vi "FTW-Container-Value-EXT.vi"(0 "JSON":refnum<class "FTW-Container.lvclass">, 11 "error in":errorcluster) -> (4 "JSON out":refnum<class "FTW-Container.lvclass">, 8 "Value":ext, 15 "error out":errorcluster)   [LabVIEW 2015, in "FTW-Container.lvclass"]
uses:
  FTW-Container.lvclass
  FTW-Container.lvclass/FTW-Container.ctl
  <vilib>/Utility/Data Type/NI_Data Type.lvlib
panel:
  # "Inputs"
  # "Outputs"
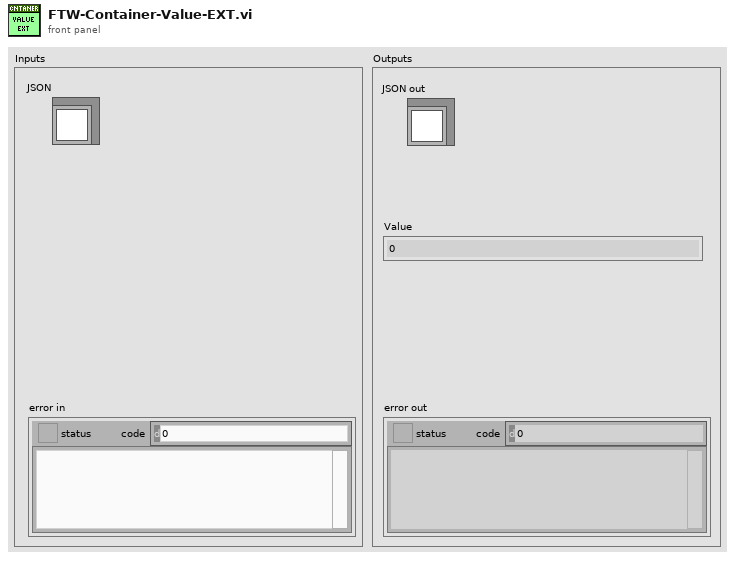
[diagram p1: front panel]
types:
  T1 = typedef "NI_Data Type.lvlib/Data Type.ctl" = enum8{"Invalid Type", "Void", "I8", "I16", "I32", "I64", "U8", "U16", "U32", "U64", "Single Float", "Double Float", "Extended Float", "Single Complex", "Double Complex", "Extended Complex", "Enum U8", "Enum U16", "Enum U32", "Enum U64", "Single Float With Unit", "Double Float With Unit", "Extended Float With Unit", "Single Complex with Unit", "Double Complex with Unit", "Extended Complex with Unit", "Boolean", "String", "Path", "Picture", "Tag", "Array", "Cluster", "Variant", "LV Variant", "Waveform", "Timestamp", "Digital Waveform", "Digital Data", "ExpressData", "Refnum", "External Data", "VI", "Poly VI", "LabVIEW Class Instance", "Fixed Point"}
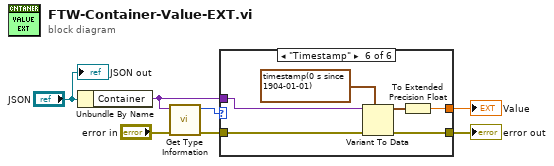
[diagram p0: block diagram]
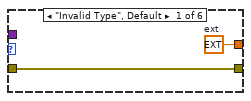
[diagram p2: hidden frame]
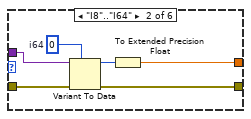
[diagram p3: hidden frame]
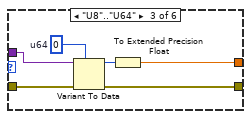
[diagram p4: hidden frame]
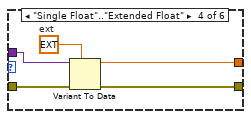
[diagram p5: hidden frame]
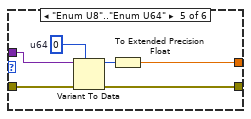
[diagram p6: hidden frame]
diagram:
  n1 = Unbundle By Name("JSON") -> ("Container"=w1:variant)
  n2 = call <vilib>:"Get Type Information.vi"("error in (no error)"="error in", "Variant"=w1) -> ("error out"=w4:errorcluster, "Type"=w3:T1)  [unwired: 5 in, 3 out]
  n3 = case shown="\"Timestamp\"" w3 {
    tunnel: w4 -> [w9 w14 w20 w25 w31 w37]
    tunnel: w1 -> [_ w13 w19 w24 w30 w36]
    tunnel: [w9 w12 w18 w23 w29 w35] -> w6
    tunnel: [w8 w10 w16 w22 w27 w33] -> w5
    frame "Invalid Type", Default {
      w8 = ext 0.0  # ext
    }
    frame "I8".."I64" {
      w15 = i64 0  # i64
      n4 = Variant To Data(error in=w14, type=w15, Variant=w13) -> (data=w11:i64, error out=w12:errorcluster)
      n5 = To Extended Precision Float(1:w11) -> (0:w10:ext)
    }
    frame "U8".."U64" {
      w21 = u64 0  # u64
      n6 = Variant To Data(error in=w20, type=w21, Variant=w19) -> (data=w17:u64, error out=w18:errorcluster)
      n7 = To Extended Precision Float(1:w17) -> (0:w16:ext)
    }
    frame "Single Float".."Extended Float" {
      w26 = ext 0.0  # ext
      n8 = Variant To Data(error in=w25, type=w26, Variant=w24) -> (data=w22:ext, error out=w23:errorcluster)
    }
    frame "Enum U8".."Enum U64" {
      w32 = u64 0  # u64
      n9 = Variant To Data(error in=w31, type=w32, Variant=w30) -> (data=w28:u64, error out=w29:errorcluster)
      n10 = To Extended Precision Float(1:w28) -> (0:w27:ext)
    }
    frame "Timestamp" {
      n11 = Variant To Data(error in=w37, type=timestamp(0 s since 1904-01-01), Variant=w36) -> (data=w34:timestamp, error out=w35:errorcluster)
      n12 = To Extended Precision Float(1:w34) -> (0:w33:ext)
    }
  }
  "error out" <- w6
  "Value" <- w5
  "JSON out" <- "JSON"
